vi "Select Products.vi"(8 "error in (no error)":errorcluster, 10 "Productos":i32(listbox), 11 "Coca Actors in":refnum<class "Coca Actors.lvclass">) -> (0 "error out":errorcluster, 3 "Coca Actors out":refnum<class "Coca Actors.lvclass">)   [LabVIEW 2020, in "Coca Actors.lvlib" / "Coca Actors.lvclass"]
uses:
  Coca Actors.lvclass
  Coca Actors.lvclass/Coca Actors.ctl
panel:
  out "output array":string[](array[string])
  in  "Data":string[](array[string])
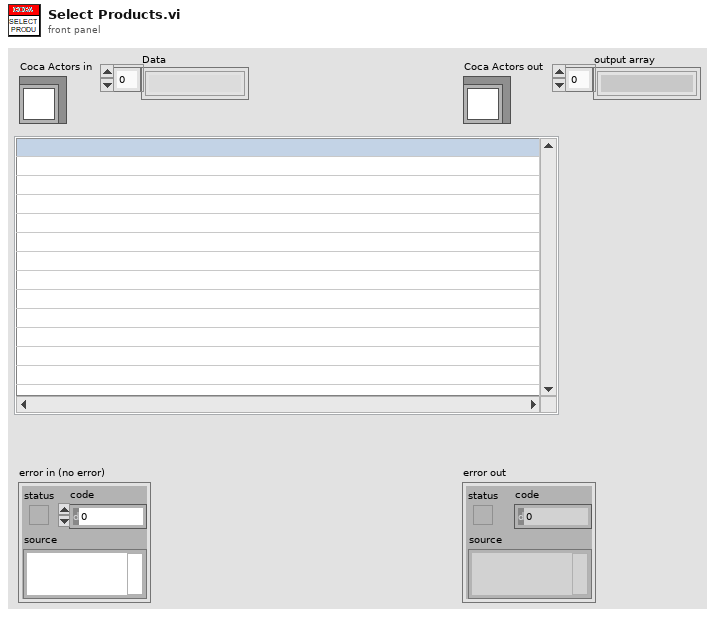
[diagram p1: front panel]
types:
  T1 = cluster{"Data[0]":string, "Data[1]":string, "Data[2]":string, "Data[3]":string, "Data[4]":string, "Data[5]":string, "Data[6]":string, "Data[7]":string, "Data[8]":string}
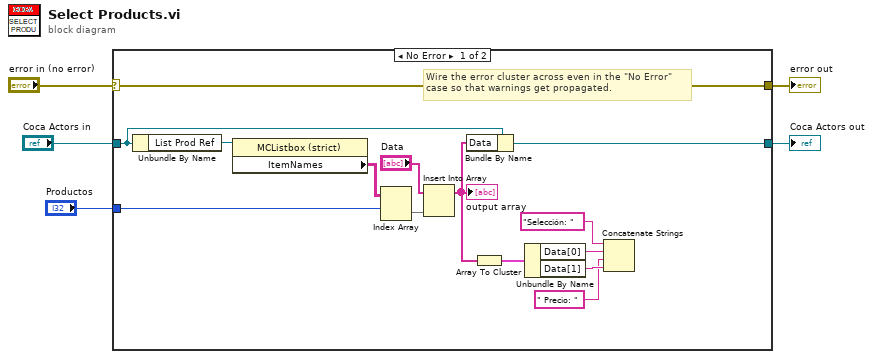
[diagram p0: block diagram]
diagram:
  n1 = case shown="No Error" "error in (no error)" {
    selector: "error in (no error)" -> [w19 w21]
    tunnel: [w19 w21] -> w4
    tunnel: [w12 w20] -> w2
    tunnel: "Coca Actors in" -> [w18 w20]
    tunnel: "Productos" -> [w15 _]
    frame No Error {
      # "Wire the error cluster across even in the \"No Error\"\ncase so that warnings get propagated."
      n2 = Unbundle By Name(w18) -> ("List Prod Ref"=w17:refnum<vi>)
      n3 = property class="MCListbox (strict)"(reference=w17) -> ("ItemNames"=w16:string[][])  [unwired: 1 in, 2 out]
      n4 = Index Array(array=w16, index (row)=w15) -> (element=w14:string[])  [unwired: 1 in]
      n5 = Insert Into Array(array="Data", new element=w14) -> (w11:string[])  [unwired: 1 in]
      "output array" <- w11
      n6 = Bundle By Name(cluster=w18, "Data"=w11) -> (w12:refnum<class "Coca Actors.lvclass">)
      n7 = Array To Cluster(array=w11) -> (cluster=w10:T1)
      n8 = Unbundle By Name(w10) -> ("Data[0]"=w9:string, "Data[1]"=w8:string)
      n9 = Concatenate Strings("Selección: " ("string"), w9, " Precio: " ("string"), w8) -> ()  [unwired: 1 out]
    }
    frame Error {
    }
  }
  "error out" <- w4
  "Coca Actors out" <- w2
